vi "tdms_write_Header.vi"() -> ()   [LabVIEW 2022 SP3]
uses:
  <vilib>/Utility/TDMS File Viewer/NI_TDMS File Viewer.lvlib
panel:
  in  "file path":path
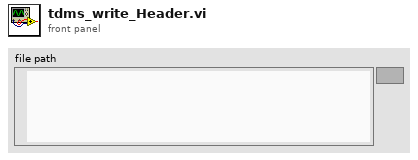
[diagram p1: front panel]
types:
  T1 = enum16{"open", "open or create", "create or replace", "create", "open (read-only)"}
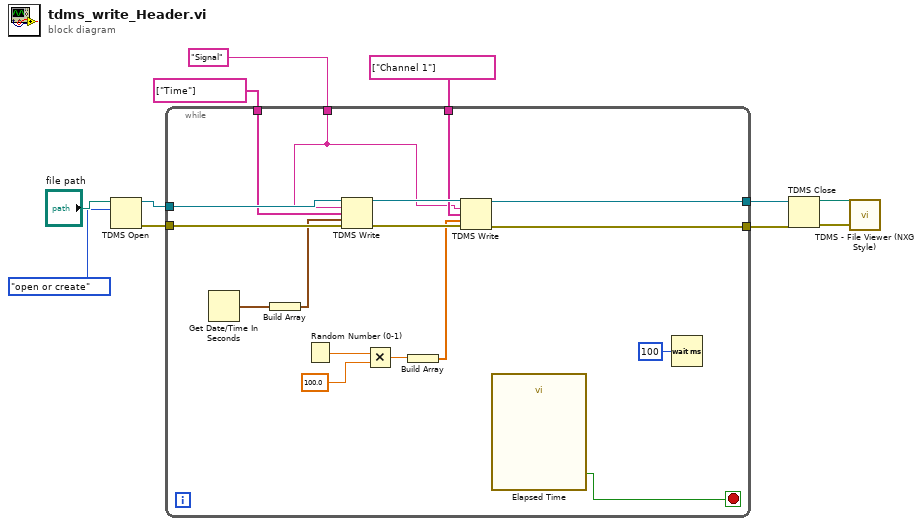
[diagram p0: block diagram]
diagram:
  n1 = TDMS Open(10:T1."open or create" ("operation (0:open)"), 11:"file path") -> (0:w8:errorcluster, 3:w9:refnum<k34>)  [unwired: 5 in]
  n2 = while {
    tunnel: w9 -> [w28]
    tunnel: w8 -> [w27]
    tunnel: "Signal" ("group name in (Untitled)") -> [w22]
    tunnel: string[] ["Time"] ("channel name(s) in (Untitled)") -> [w26]
    tunnel: string[] ["Channel 1"] ("channel name(s) in (Untitled)") -> [w23]
    tunnel: [w14] -> w4
    tunnel: [w13] -> w3
    stop <- w12 stop-if-true
    n3 = Get Date/Time In Seconds() -> (seconds since 1Jan1904=w21:timestamp)
    n4 = Build Array "Build Array"(w21) -> (w20:timestamp[])
    n5 = Random Number (0-1)() -> (number: 0 to 1=w19:dbl)
    n6 = TDMS Write(0:w28, 5:w22, 7:w26, 9:w20, 11:w27) -> (4:w25:refnum<k34>, 15:w24:errorcluster)  [unwired: 1 in, 2 out]
    n7 = Multiply(x=w19, y=100.0) -> (x*y=w17:dbl)
    n8 = Build Array(w17) -> (w16:dbl[])
    n9 = TDMS Write(0:w25, 5:w22, 7:w23, 9:w16, 11:w24) -> (4:w14:refnum<k34>, 15:w13:errorcluster)  [unwired: 1 in, 2 out]
    n10 = call "Elapsed Time"() -> ("Time has Elapsed"=w12:bool)  [unwired: 12 in, 7 out]
    n11 = Wait (ms)(milliseconds to wait=u32 100) -> ()  [unwired: 1 out]
  }
  n12 = TDMS Close(8:w3, 11:w4) -> (0:w1:errorcluster, 3:w2:path)
  n13 = call <vilib>:"TDMS - File Viewer (NXG Style).vi"("error in"=w1, "file in"=w2) -> ()  [unwired: 8 in, 2 out]
